vi "KalibrationLog.vi"(7 "HM-Nr 2":string, 8 "error in (no error)":errorcluster, 9 "Sensetivity mV/Pa":string, 10 "nominal Frequency/Hz":string, 11 "nominal Level/dBSpl":string) -> (0 "error IO":errorcluster)   [LabVIEW 2018]
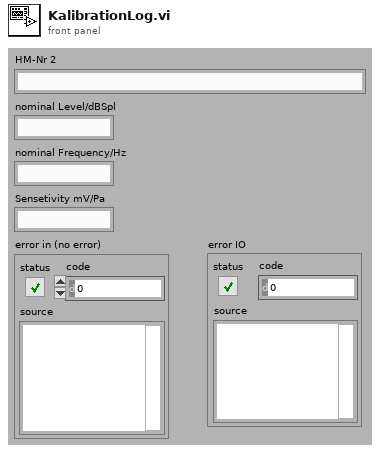
[diagram p1: front panel]
types:
  T1 = enum16{"open", "replace", "create", "open or create", "replace or create", "replace or create with confirmation"}
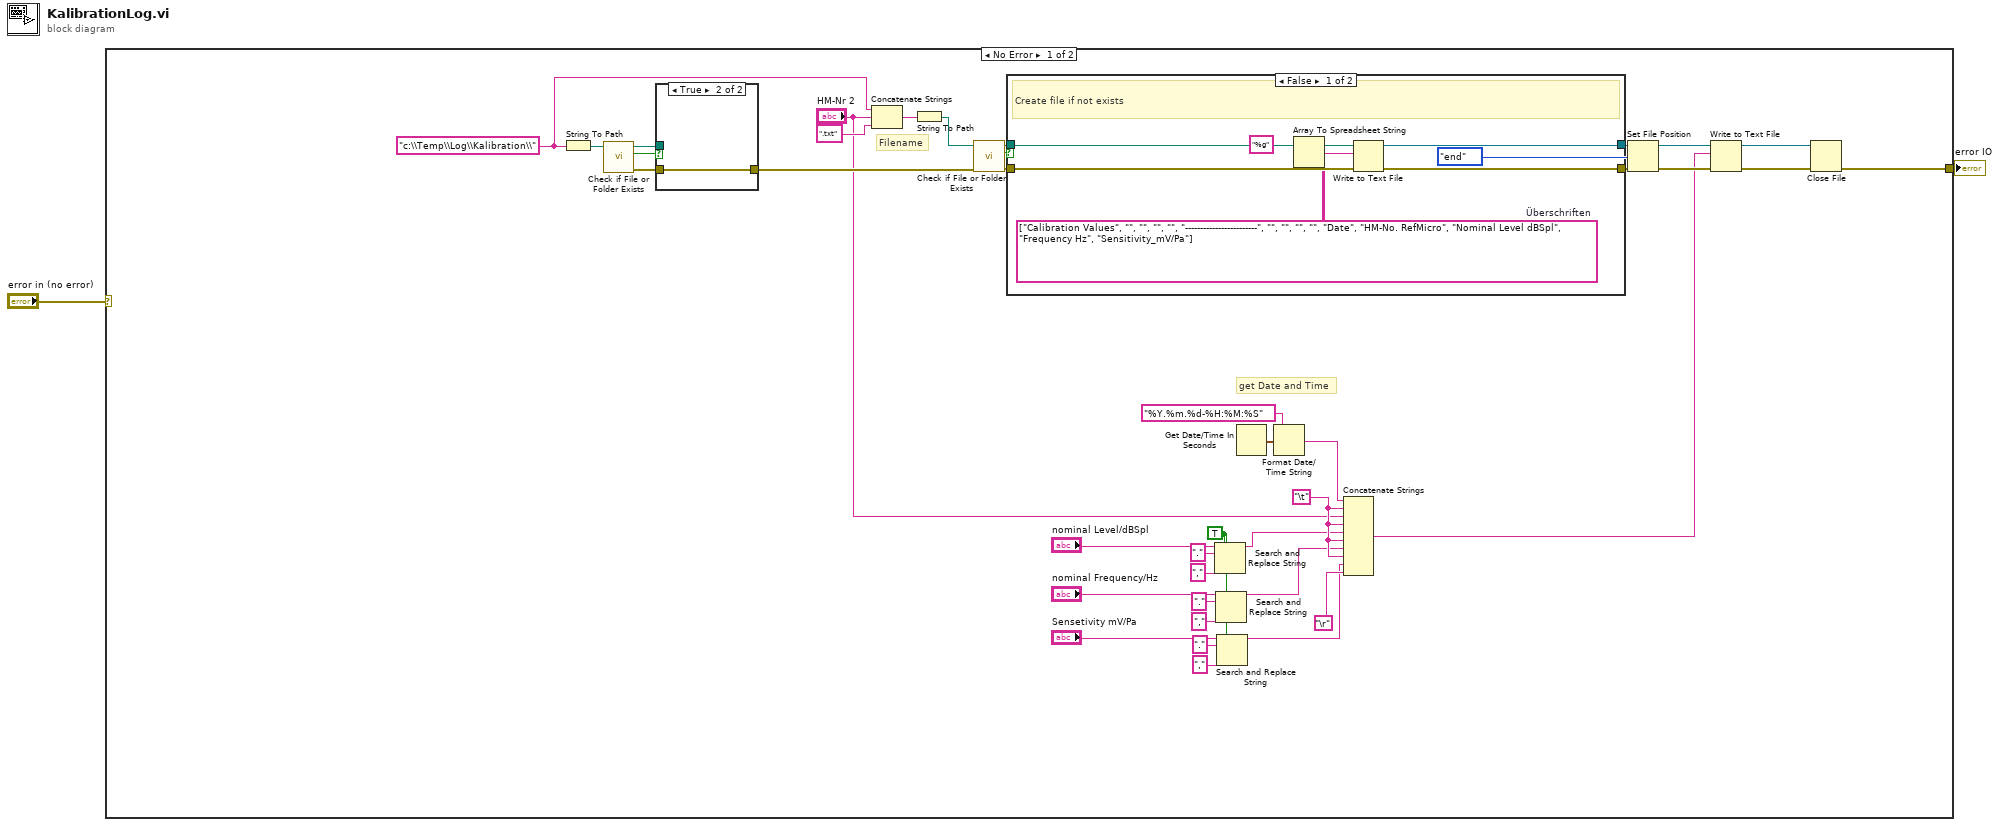
[diagram p0: block diagram]
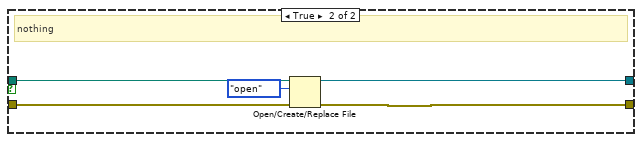
[diagram p2: hidden frame]
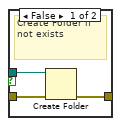
[diagram p3: hidden frame]
diagram:
  n1 = case shown="No Error" "error in (no error)" {
    selector: "error in (no error)" -> [_ w59]
    tunnel: [w22 w59] -> w2
    frame No Error {
      w9 = TRUE ("replace all? (F)")
      w17 = "\t"
      w33 = "c:\\Temp\\Log\\Kalibration\\" ("string")
      # "Filename"
      # "get Date and Time"
      n2 = String To Path(string=w33) -> (path=w37:path)
      n3 = call <vilib>:"Check if File or Folder Exists.vi"("path"=w37) -> ("error out"=w40:errorcluster, "file or folder exists?"=w39:bool, "dup path"=w38:path)  [unwired: 8 in]
      n4 = case shown="True" w39 {
        tunnel: w40 -> [w57 w58]
        tunnel: [w56 w58] -> w32
        tunnel: w38 -> [w55 _]
        frame False {
          # "Create Folder if not exists"
          n5 = Create Folder(path (use dialog)=w55, error in=w57) -> (error out=w56:errorcluster)  [unwired: 1 in, 2 out]
        }
        frame True {
        }
      }
      n6 = Concatenate Strings(w33, "HM-Nr 2", ".txt" ("string")) -> (w35:string)
      n7 = String To Path(string=w35) -> (path=w34:path)
      n8 = call <vilib>:"Check if File or Folder Exists.vi"("error in (no error)"=w32, "path"=w34) -> ("error out"=w31:errorcluster, "file or folder exists?"=w29:bool, "dup path"=w30:path)  [unwired: 7 in]
      n9 = case shown="False" w29 {
        tunnel: [w44 w51] -> w28
        tunnel: w31 -> [w49 w52]
        tunnel: w30 -> [w48 w54]
        tunnel: [w43 w53] -> w27
        frame False {
          w47 = string[][] [["Calibration Values", "", "", "", ""], ["------------------------", "", "", "", ""], ["Date", "HM-No. RefMicro", "Nominal Level dBSpl", "Frequency Hz", "Sensitivity_mV/Pa"]]  # Überschriften
          # "Create file if not exists"
          n10 = Array To Spreadsheet String(array=w47, 3:"%g" ("Format-String")) -> (spreadsheet string=w45:string)  [unwired: 1 in]
          n11 = Write to Text File(file (use dialog)=w48, text=w45, error in=w49) -> (refnum out=w43:refnum<file>, error out=w44:errorcluster)  [unwired: 1 in, 1 out]
        }
        frame True {
          # "nothing"
          n12 = Open/Create/Replace File(file path (use dialog)=w54, error in=w52, operation (0:open)=T1."open") -> (refnum out=w53:refnum<file>, error out=w51:errorcluster)  [unwired: 3 in, 1 out]
        }
      }
      n13 = Search and Replace String(replace all?=w9, input string="nominal Level/dBSpl", search string=".", replace string="," ("replace string (\"\")")) -> (result string=w5:string)  [unwired: 4 in, 3 out]
      n14 = Search and Replace String(replace all?=w9, input string="nominal Frequency/Hz", search string=".", replace string="," ("replace string (\"\")")) -> (result string=w4:string)  [unwired: 4 in, 3 out]
      n15 = Search and Replace String(replace all?=w9, input string="Sensetivity mV/Pa", search string=".", replace string="," ("replace string (\"\")")) -> (result string=w3:string)  [unwired: 4 in, 3 out]
      n16 = Get Date/Time In Seconds() -> (seconds since 1Jan1904=w42:timestamp)
      n17 = Format Date/Time String(time format string (%c)="%Y.%m.%d-%H:%M:%S", seconds (now)=w42) -> (date/time string=w20:string)  [unwired: 1 in]
      n18 = Concatenate Strings(w20, w17, "HM-Nr 2", w17, w5, w17, w4, w17, w3, "\r") -> (w18:string)
      n19 = Set File Position(refnum=w27, from (0:start)=enum16{"start", "end", "current"}."end", error in=w28) -> (refnum out=w25:refnum<file>, error out=w24:errorcluster)  [unwired: 1 in]
      n20 = Write to Text File(file (use dialog)=w25, text=w18, error in=w24) -> (refnum out=w21:refnum<file>, error out=w23:errorcluster)  [unwired: 1 in, 1 out]
      n21 = Close File(refnum=w21, error in=w23) -> (error out=w22:errorcluster)  [unwired: 1 out]
    }
    frame Error {
    }
  }
  "error IO" <- w2
